vi "Trigger Setup.vi"(6 "Delay Value (s) (0.0)":dbl min=0.0 max=6.0 step=0.1 format="%.4f", 7 "Trigger Source (0: Internal)":u32(slide) max=3 step=1, 8 "error in (no error)":errorcluster, 10 "Cont (F: Off)":bool, 11 "VISA resource name":refnum<visa-resource-name>) -> (0 "error out":errorcluster, 3 "VISA resource name out":refnum<visa-resource-name>)   [LabVIEW 2015, in "Agilent 428X Series.lvlib"]
doc: "This function sets the trigger system to the continuous ON or OFF condition and sets the Trigger source. In the continuous ON condition, after reading the measurement data by a controller, the IDDLE STATE is automatically set to the WAIT FOR TRIGGER STATE."
uses:
  Agilent 428X Series.lvlib
panel:
  # "On\nOff"
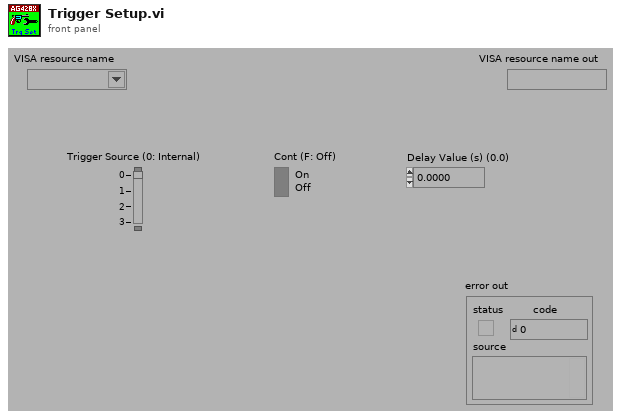
[diagram p1: front panel]
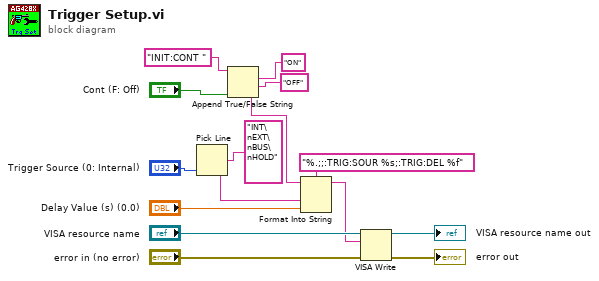
[diagram p0: block diagram]
diagram:
  n1 = Pick Line(multi-line string="INT\nEXT\nBUS\nHOLD", line index="Trigger Source (0: Internal)") -> (output string=w3:string)  [unwired: 1 in]
  n2 = Append True/False String(1:"Cont (F: Off)", 2:"OFF", 3:"ON", 4:"INIT:CONT ") -> (0:w2:string)
  n3 = Format Into String(format string="%.;;:TRIG:SOUR %s;:TRIG:DEL %f", initial string=w2, w3, "Delay Value (s) (0.0)") -> (resulting string=w1:string)  [unwired: 1 in, 1 out]
  n4 = VISA Write(VISA resource name="VISA resource name", write buffer=w1, error in (no error)="error in (no error)") -> (VISA resource name out=→"VISA resource name out":refnum<visa-resource-name>, error out=→"error out":errorcluster)  [unwired: 1 out]
